vi "EX 6-3 IR Sensor.vi"() -> ()   [LabVIEW 2011, in "LabVIEW Interface for Arduino.lvlib"]
doc: "An example that uses the Arduino with a IR sensor to detect movement. The example triggers an action when movement is seen and when movement stops being seen. The user can set a threshold for the number of seconds movement must be seen to trigger a movement action."
uses:
  <vilib>/LabVIEW Interface for Arduino/LabVIEW Interface for Arduino.lvlib
panel:
  in  "Stop":bool
  in  "Movement Limit (seconds)":dbl
  out "Movement Stopped Action":bool
  out "Movement Started Action":bool
  out "Movement Seen For(seconds)":dbl
  out "LastMovement":timestamp
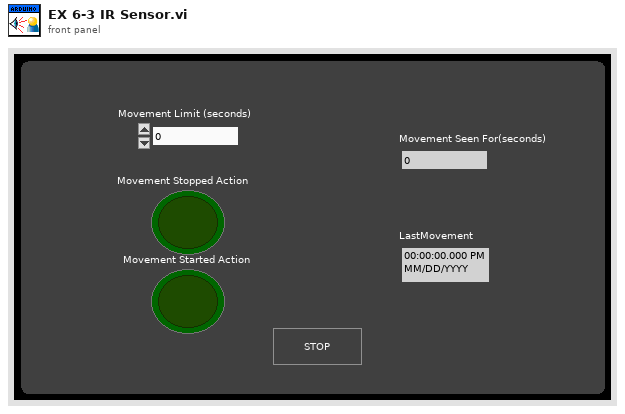
[diagram p1: front panel]
types:
  T1 = typedef "LabVIEW Interface for Arduino.lvlib/Arduino Resource.ctl" = cluster{"VISA resource":refnum<visa-resource-name>, "Board Type":T2, "Connection Type":enum8{"USB / Serial"}, "Bytes Per Packet (15)":u8}
  T2 = typedef "LabVIEW Interface for Arduino.lvlib/Board Type.ctl" = enum16{"Uno", "Dimuelanove w/Atmega 328", "Mega 2560"}
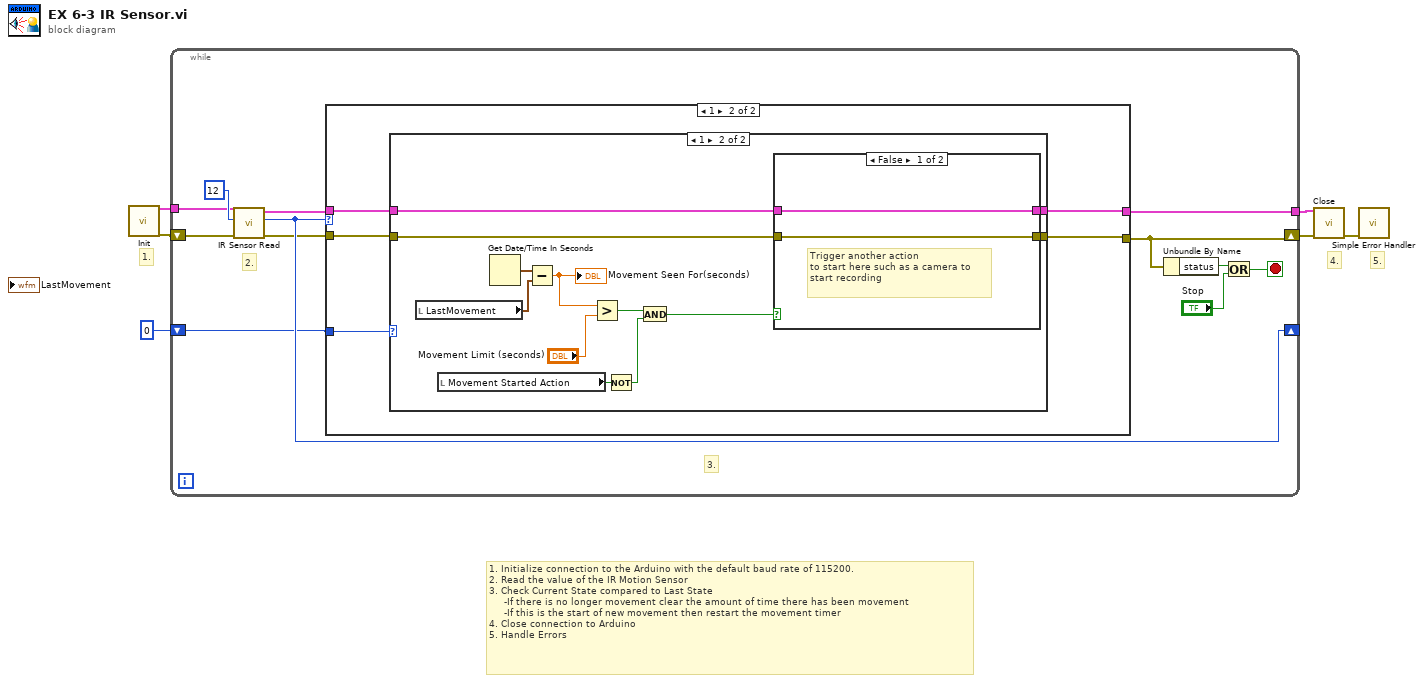
[diagram p0: block diagram]
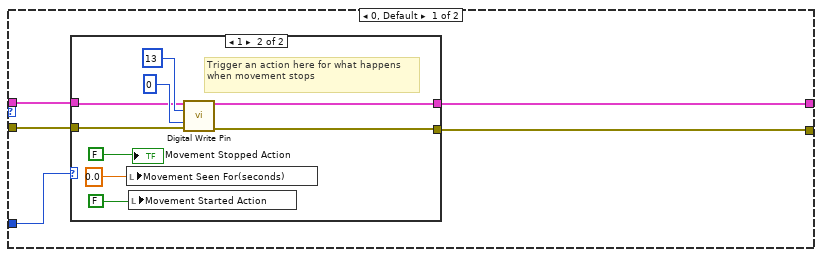
[diagram p2: hidden frame]
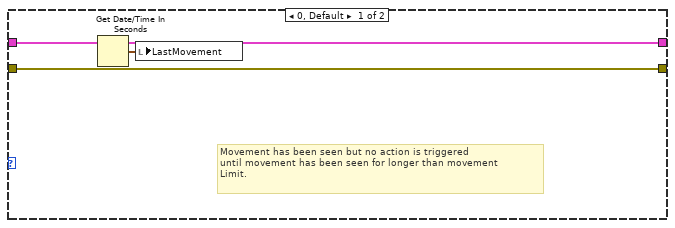
[diagram p4: hidden frame]
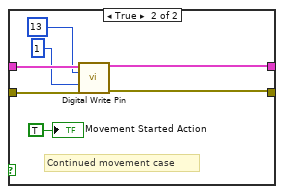
[diagram p5: hidden frame]
diagram:
  # "5."
  # "4."
  # "1."
  # "1. Initialize connection to the Arduino with the default baud rate of 115200.\n2. Read the value of the IR Motion Sensor\n3. Check Current State compared to Last State\n     -If there is no longer movement clear the amount of time there has been movement\n     -If this is the start of new movement then restart the movement timer\n4. Close connection to Arduino\n5. Handle Errors"
  n1 = call <vilib>:"Init.vi"() -> ("Arduino Resource"=w4:T1, "error out"=w6:errorcluster)  [unwired: 18 in]
  n2 = while {
    shift-right: [w7] -> w5
    shift-left: w6 -> [w17]
    tunnel: w4 -> [w12]
    shift-right: [w14] -> _
    shift-left: u8 0 ("MotionDetected") -> [w13]
    tunnel: [w10] -> w2
    stop <- w15 stop-if-true
    # "3."
    # "2."
    n3 = call <vilib>:"IR Sensor Read.vi"("error in"=w17, "Sensor Pin"=u8 12 ("Select DI Pin"), "Arduino Resource"=w12) -> ("error out"=w11:errorcluster, "MotionDetected"=w14:u8, "Arduino Resource"=w9:T1)  [unwired: 6 in]
    n4 = case shown="1" w14 {
      tunnel: w13 -> [w23 w39]
      tunnel: w11 -> [w22 w36]
      tunnel: [w21 w35] -> w7
      tunnel: [w20 w37] -> w10
      tunnel: w9 -> [w19 w38]
      frame 0, Default {
        n5 = case shown="1" w23 {
          tunnel: w22 -> [w24 w30]
          tunnel: [w24 w29] -> w21
          tunnel: [w25 w27] -> w20
          tunnel: w19 -> [w25 w26]
          frame 0, Default {
          }
          frame 1 {
            # "Trigger an action here for what happens\nwhen movement stops"
            n6 = local write "Movement Seen For(seconds)"(0.0 ("high for")) -> ()
            n7 = local write "Movement Started Action"(FALSE ("MovementStartedAction")) -> ()
            n8 = call <vilib>:"Digital Write Pin.vi"("Arduino Resource"=w26, "Digital I/O Pin (0)"=u8 13, "Value (0)"=u8 0, "error in"=w30) -> ("Arduino Resource"=w27:T1, "error out"=w29:errorcluster)  [unwired: 10 in]
            "Movement Stopped Action" <- FALSE ("MovementStoppedAction")
          }
        }
      }
      frame 1 {
        n9 = case shown="1" w39 {
          tunnel: w38 -> [w41 w46]
          tunnel: [w41 w45] -> w37
          tunnel: w36 -> [w40 w44]
          tunnel: [w40 w43] -> w35
          frame 0, Default {
            # "Movement has been seen but no action is triggered\nuntil movement has been seen for longer than movement\nLimit."
            n10 = Get Date/Time In Seconds() -> (seconds since 1Jan1904=w42:timestamp)
            n11 = local write "LastMovement"(w42) -> ()
          }
          frame 1 {
            n12 = local read "LastMovement"() -> (w53:timestamp)
            n13 = local read "Movement Started Action"() -> (w49:bool)
            n14 = Get Date/Time In Seconds() -> (seconds since 1Jan1904=w54:timestamp)
            n15 = Subtract(x=w54, y=w53) -> (x-y=w52:dbl)
            "Movement Seen For(seconds)" <- w52
            n16 = Greater?(x=w52, y="Movement Limit (seconds)") -> (0:w48:bool)
            n17 = Not(x=w49) -> (.not. x?=w50:bool)
            n18 = And(x=w48, y=w50) -> (x .and. y?=w47:bool)
            n19 = case shown="False" w47 {
              tunnel: w46 -> [w56 w62]
              tunnel: [w56 w61] -> w45
              tunnel: w44 -> [w55 w60]
              tunnel: [w55 w57] -> w43
              frame False {
                # "Trigger another action \nto start here such as a camera to\nstart recording"
              }
              frame True {
                # "Continued movement case"
                n20 = call <vilib>:"Digital Write Pin.vi"("Arduino Resource"=w62, "Digital I/O Pin (0)"=u8 13, "Value (0)"=u8 1, "error in"=w60) -> ("Arduino Resource"=w61:T1, "error out"=w57:errorcluster)  [unwired: 10 in]
                "Movement Started Action" <- TRUE ("MovementStartedAction")
              }
            }
          }
        }
      }
    }
    n21 = Unbundle By Name(w7) -> ("status"=w16:bool)
    n22 = Or(x=w16, y="Stop") -> (x .or. y?=w15:bool)
  }
  n23 = call <vilib>:"Close.vi"("Arduino Resource"=w2, "error in"=w5) -> ("error out"=w3:errorcluster)  [unwired: 13 in]
  n24 = call <vilib>:"Simple Error Handler.vi"("error in (no error)"=w3) -> ()  [unwired: 4 in, 5 out]
